vi "test_414.vi"() -> ()   [LabVIEW 2009]
uses:
  OGRE/nick/FPGA/behaviors/driveable paths/test variable.vi
  <vilib>/Platform/TimedLoop/XDataNode/XDataNode.xnode
  <vilib>/Platform/TimedLoop/XDataNode/timing_clust.ctl
  <vilib>/Platform/TimedLoop/XDataNode/XDNodeRunTimeDep.lvlib
  <vilib>/Platform/TimedLoop/XDataNode/wakeup.ctl
  <vilib>/Platform/TimedLoop/XDataNode/nitl_modes.ctl
  <vilib>/Platform/TimedLoop/XDataNode/loadlvalarms.vi
panel:
  out "XY Graph 2":cluster{"Y":dbl[], "Y":dbl[]}[](graph)
  in  "x LIDAR position":i16
  in  "y LIDAR position":i16
  out "Y positions":i16[](array[numeric])
  out "x positions":i16[](array[numeric])
  in  "number 16\" iterations":i32
  out "XY Graph":cluster{"Y":dbl[], "Y":dbl[]}[](graph)
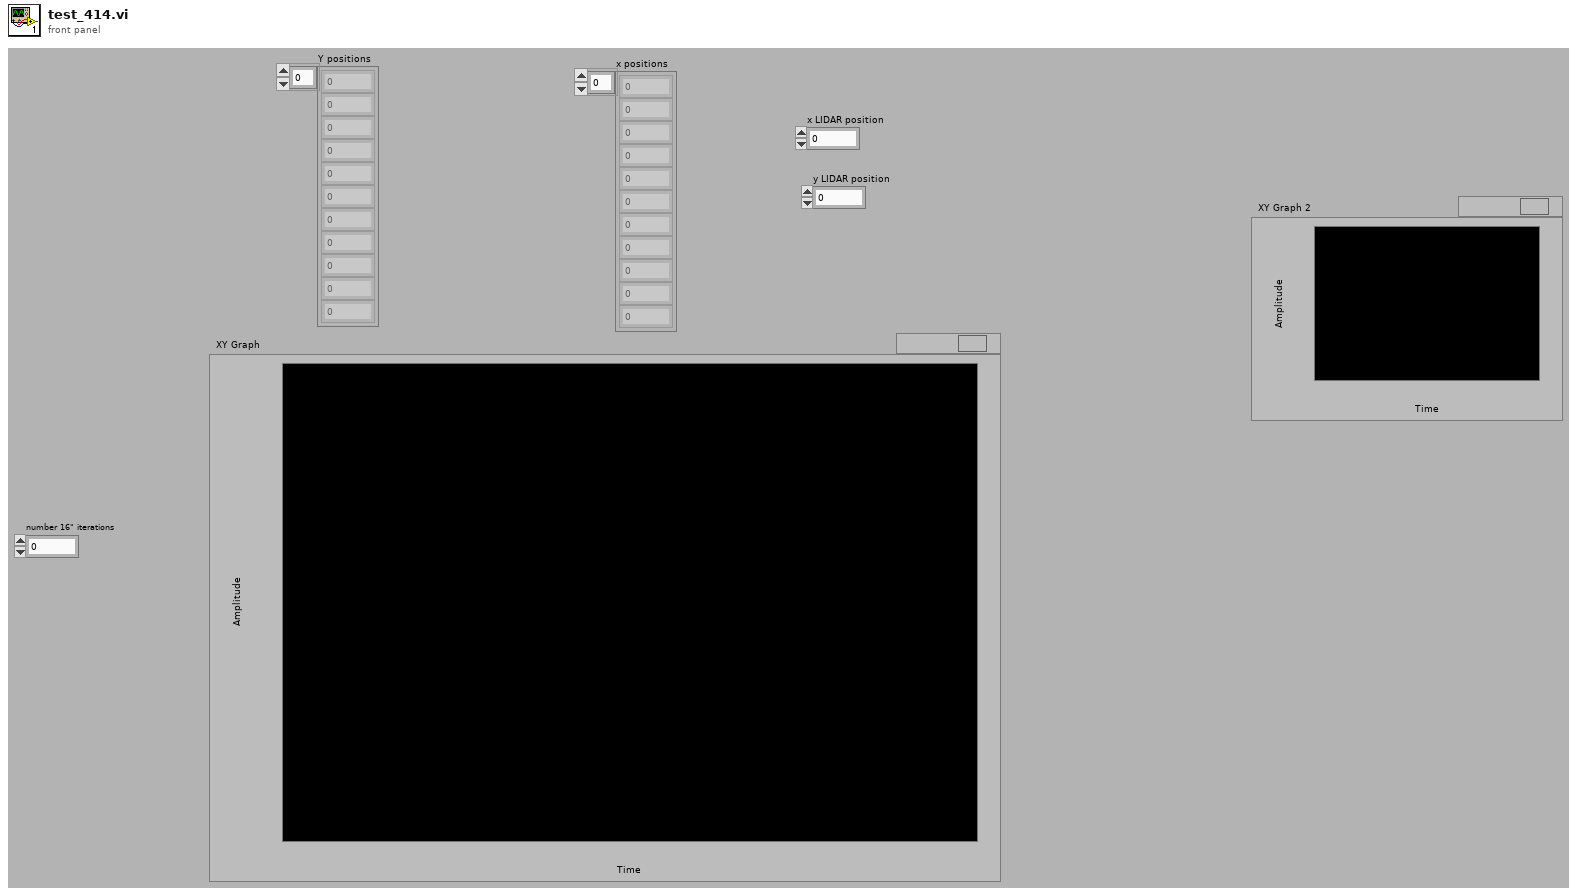
[diagram p1: front panel]
types:
  T1 = typedef "XDNodeRunTimeDep.lvlib/timing_clust.ctl" = cluster{"Expected End [f-1]":u64, "Actual End [f-1]":u64, "Finished Late? [f-1]":bool, "Expected End [i-1]":u64, "Actual End [i-1]":u64, "Finished Late? [i-1]":bool, "Expected Start [i]":u64, "Actual Start [i]":u64, "Expected Start [f]":u64, "Actual Start [f]":u64, "Source Name":string, "Structure Name":string, "Period":i64, "Deadline":i64, "Offset":i64, "Start":i64, "Priority":i32, "Timeout":i32, "Mode":T2, "Wakeup Reason":T3, "Error":errorcluster, "Source Type":string, "Secondary Source Type":string, "Global End Time":u64, "Global Start Time":u64, "Frame Duration":u64, "Iteration Duration":u64, "Assigned CPU":i32, "I/O Scan Engine Mode":u32}
  T2 = typedef "XDNodeRunTimeDep.lvlib/nitl_modes.ctl" = enum32{"No Change", "Process missed periods, maintain original phase", "Discard missed periods, maintain original phase", "Process missed periods, ignore original phase", "Discard missed periods, ignore original phase"}
  T3 = typedef "XDNodeRunTimeDep.lvlib/wakeup.ctl" = enum32{"Normal", "Aborted", "Asynchronous wakeup", "Timing source error", "Timed loop error", "Timeout"}
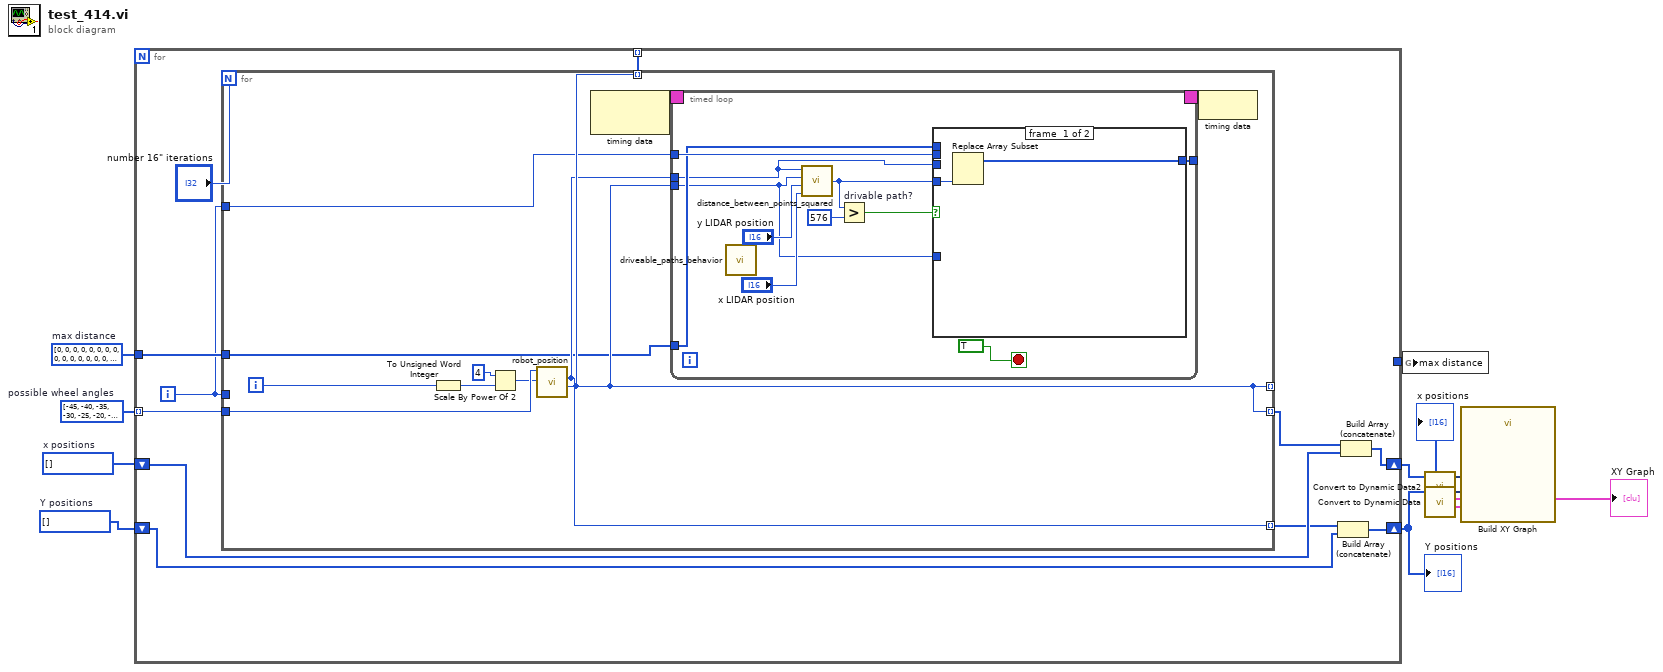
[diagram p0: block diagram]
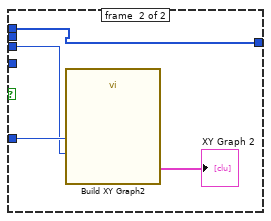
[diagram p2: hidden frame]
diagram:
  w5 = i16[] []  # Y positions
  w6 = i16[] []  # x positions
  w8 = i8[] [-45, -40, -35, -30, -25, -20, -15, -10, -5, 0, 5, 10, 15, 20, 25, 30, 35, 40, 45]  # possible wheel angles
  w9 = i16[] [0, 0, 0, 0, 0, 0, 0, 0, 0, 0, 0, 0, 0, 0, 0, 0, 0, 0, 0]  # max distance
  n1 = for {
    tunnel: w9 -> [w21]
    tunnel: w8 -> [w13] mode=indexing
    tunnel: [_] -> w7
    shift-right: [w17] -> w2
    shift-left: w6 -> [w18]
    shift-right: [w16] -> w4
    shift-left: w5 -> [w14]
    tunnel: [w12] -> _ mode=indexing
    i -> [w11]
    n2 = for {
      N: "number 16\" iterations" -> [_]
      tunnel: w21 -> [w22]
      tunnel: w11 -> [_]
      tunnel: w13 -> [w31]
      tunnel: [w25] -> _ mode=indexing
      tunnel: [w25] -> w19 mode=indexing
      tunnel: [w24] -> w15 mode=indexing
      tunnel: [w25] -> w12 mode=indexing
      tunnel: w11 -> [w23]
      i -> [w32]
      n3 = To Unsigned Word Integer(number=w32) -> (unsigned 16bit integer=w29:u16)
      n4 = Scale By Power Of 2(n=u16 4, x=w29) -> (x*2^n=w28:u16)
      n5 = call "robot_position.vi"("Distance Along Arc"=w28, "Wheel Angle"=w31) -> ("New X Position"=w25:i8, "New Y Position"=w24:i8)  [unwired: 7 in, 1 out]
      n6 = node-c288() -> (w27:T1)  [unwired: 1 in]
      n7 = timed-loop {
        timing: w27 -> [_]
        timing-out: [_] -> w26
        tunnel: [w43] -> _
        tunnel: w24 -> [w33]
        tunnel: w25 -> [w34]
        tunnel: w23 -> [w36]
        tunnel: w22 -> [w35]
        stop <- TRUE stop-if-true
        n8 = call "distance_between_points_squared.vi"("x LIDAR position"="x LIDAR position", "y LIDAR position"="y LIDAR position", "x position"=w34, "y position"=w33) -> ("distance squared"=w38:i16)  [unwired: 2 in]
        n9 = Greater? "drivable path?"(x=w38, y=i16 576) -> (0:w39:bool)
        n10 = case shown="True" w39 {
          tunnel: w38 -> [w45 _]
          tunnel: [w44 w49] -> w43
          tunnel: w36 -> [_ _]
          tunnel: w35 -> [_ w49]
          tunnel: w34 -> [_ w48]
          tunnel: w33 -> [_ w47]
          frame #0 {
            n11 = Replace Array Subset(new element=w45) -> (w44:i16[])  [unwired: 2 in]
          }
          frame #1 {
            n12 = call "Build XY Graph2"("Y Input"=w47, "X Input"=w48) -> ("XY Graph"=→"XY Graph 2":cluster{"Y":dbl[], "Y":dbl[]}[])  [unwired: 8 in, 1 out]
          }
        }
      }
      n13 = node-c288(w26) -> ()
    }
    n14 = Build Array (concatenate)(w15, w14) -> (w16:i16[])
    n15 = Build Array (concatenate)(w19, w18) -> (w17:i16[])
  }
  "x positions" <- w2
  "Y positions" <- w4
  n16 = call "driveable_paths_behavior.vi"() -> ()  [unwired: 1 in]
  n17 = global write "test variable.vi" "max distance"(w7) -> ()
  n18 = call "Convert to Dynamic Data2"("Array"=w2) -> ("Dynamic Data Type"=w1:dynamicdata)  [unwired: 3 in]
  n19 = call "Convert to Dynamic Data"("Array"=w4) -> ("Dynamic Data Type"=w3:dynamicdata)  [unwired: 3 in]
  n20 = call "Build XY Graph"("Y Input"=w3, "X Input"=w1) -> ("XY Graph"=→"XY Graph":cluster{"Y":dbl[], "Y":dbl[]}[])  [unwired: 8 in, 1 out]
